vi "PLL_PID.vi"(8 "error in (no error)":errorcluster, 11 "DSP.lvclass":refnum<class "DSP.lvclass">) -> (0 "error out":errorcluster, 2 "phase out":dbl, 3 "DSP.lvclass":refnum<class "DSP.lvclass">)   [LabVIEW 2019, in "DSP.lvclass"]
uses:
  DSP.lvclass
  DSP.lvclass/DSP.ctl
  <vilib>/Analysis/baseanly.llb/Mean (DBL).vi
  <vilib>/addons/control/pid/pid.llb/PID (DBL).vi
  <vilib>/addons/control/pid/NI_PID_pid.lvlib
  <vilib>/Analysis/NI_AALBase.lvlib
panel:
  in  "x":dbl=4.77
  in  "mean?":bool
  out "TC (s)":dbl
  out "frequency (Hz)":dbl
  in  "PID gains (Phase)":T1={"proportional gain (Kc)"=-1.0, "integral time (Ti, min)"=0.025, "derivative time (Td, min)"=0.0} {"derivative time (Td, min)" format="%.3f"; "integral time (Ti, min)" format="%.3f"; "proportional gain (Kc)" format="%.3f"}
  out "Waveform Chart":T2(graph)
  # "4.77"
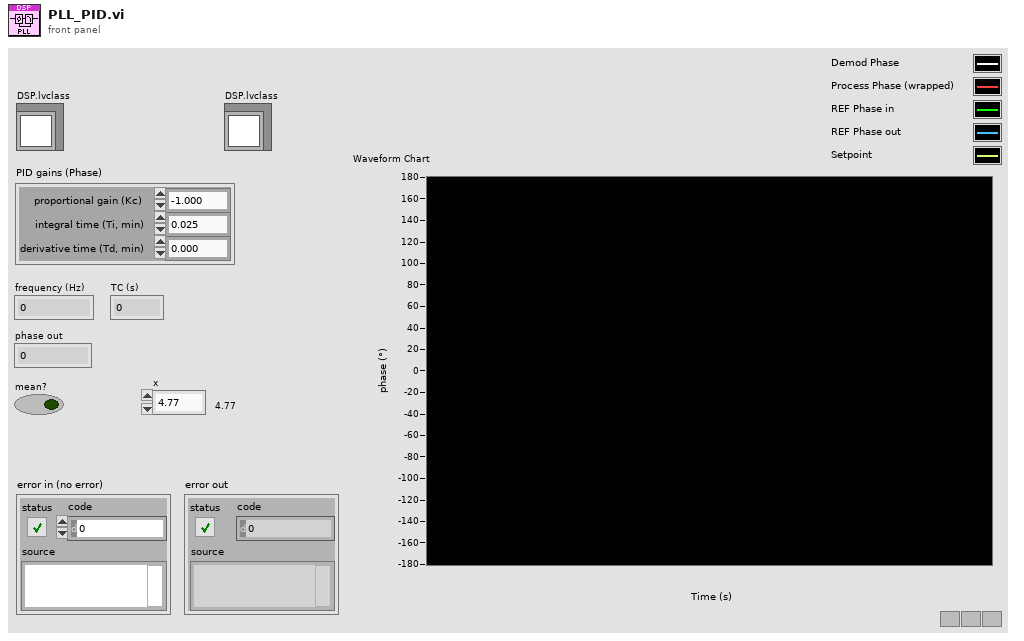
[diagram p1: front panel]
types:
  T1 = cluster{"proportional gain (Kc)":dbl, "integral time (Ti, min)":dbl, "derivative time (Td, min)":dbl}
  T2 = cluster{"value":dbl, "wrapped phase":dbl, "Phase":dbl, "wrapped phase":dbl, "setpoint":dbl}
  T3 = typedef "DSP.lvclass/REF.Channel--Cluster--Array.ctl" = T4[]
  T4 = typedef "DSP.lvclass/REF.Channel--Cluster.ctl" = cluster{"Enable?":bool, "Channel":i32, "Frequency":dbl, "Phase":dbl, "TC":dbl, "Roll-Off":i32}
  T5 = cluster{"value":dbl, "wrapped phase":dbl, "Phase":dbl, "wrapped phase":dbl, "setpoint":dbl}[]
  T6 = cluster{"filter structure":enum32{"IIR 2nd Order", "IIR 4th Order"}, "Reverse Coefficients":dbl[], "Forward Coefficients":dbl[]}[]
  T7 = cluster{dbl, "wrapped phase":dbl, "Phase":dbl, "wrapped phase":dbl, "setpoint":dbl}
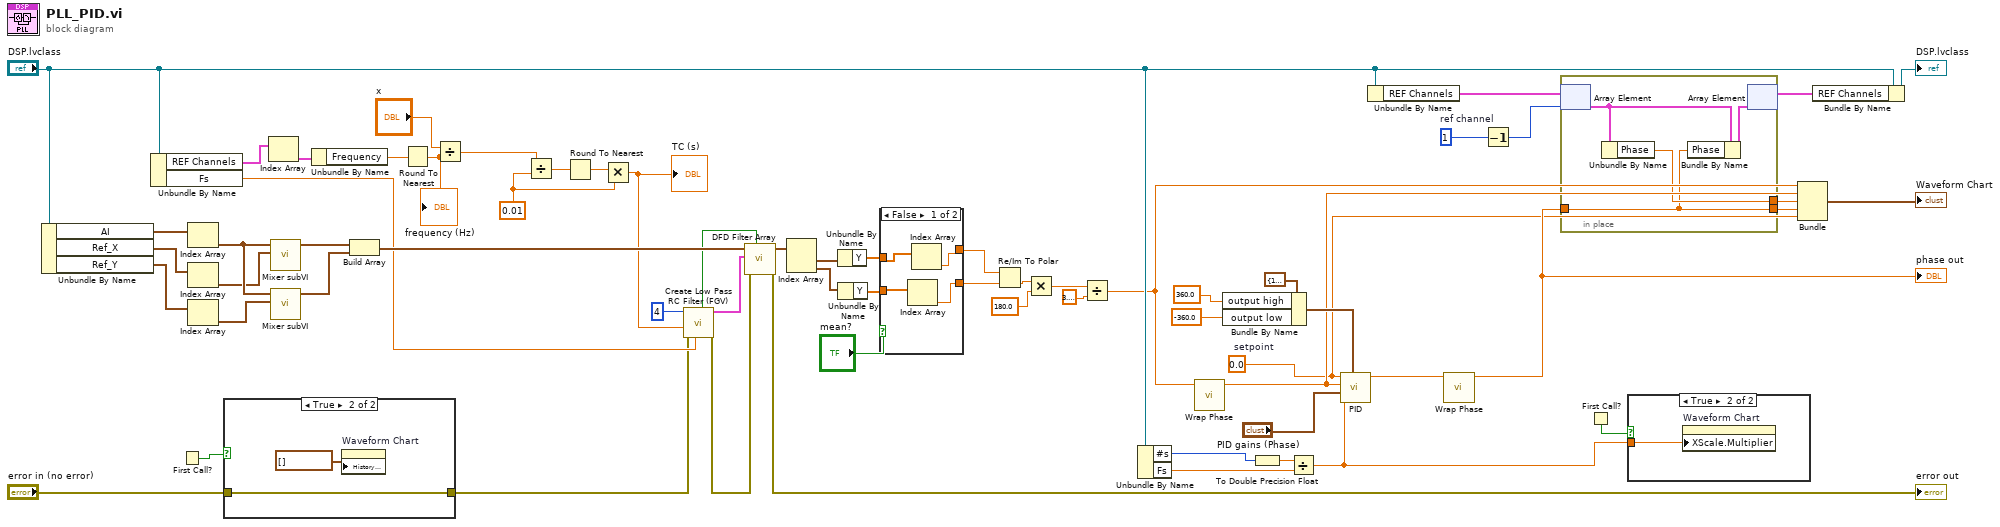
[diagram p0: block diagram]
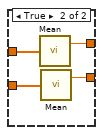
[diagram p2: hidden frame]
diagram:
  w2 = 0.01 ("y")
  w60 = 1  # ref channel
  w43 = 0.0  # setpoint
  n1 = Unbundle By Name("DSP.lvclass") -> ("AI"=w19:waveform(dbl)[], "Ref_X"=w17:waveform(dbl)[], "Ref_Y"=w16:waveform(dbl)[])
  n2 = Unbundle By Name("DSP.lvclass") -> ("REF Channels"=w36:T3, "Fs"=w37:dbl)
  n3 = First Call?() -> (First Call?: T/F=w46:bool)
  n4 = Index Array(array=w19) -> (element=w18:waveform(dbl))  [unwired: 1 in]
  n5 = Index Array(array=w17) -> (element=w15:waveform(dbl))  [unwired: 1 in]
  n6 = Index Array(array=w16) -> (element=w14:waveform(dbl))  [unwired: 1 in]
  n7 = case shown="True" w46 {
    tunnel: "error in (no error)" -> [w65 w66]
    tunnel: [w65 w66] -> w12
    frame False {
    }
    frame True {
      n8 = property on="Waveform Chart" class="WFChart (strict)"("History Data"=T5 []) -> ()  [unwired: 2 in, 2 out]
    }
  }
  n9 = Index Array(array=w36) -> (element=w35:T4)  [unwired: 1 in]
  n10 = call "Mixer subVI.vi"("Reference in"=w15, "Signal in"=w18) -> ("Signal*Reference out"=w41:waveform(dbl))  [unwired: 9 in]
  n11 = call "Mixer subVI.vi"("Reference in"=w14, "Signal in"=w18) -> ("Signal*Reference out"=w32:waveform(dbl))  [unwired: 9 in]
  n12 = Unbundle By Name(w35) -> ("Frequency"=w30:dbl)
  n13 = Build Array(w41, w32) -> (w40:waveform(dbl)[])
  n14 = Round To Nearest(number=w30) -> (nearest integer value=w29:dbl)
  "frequency (Hz)" <- w29
  n15 = Divide(x="x", y=w29) -> (x/y=w5:dbl)
  n16 = Divide(x=w5, y=w2) -> (x/y=w4:dbl)
  n17 = Round To Nearest(number=w4) -> (nearest integer value=w3:dbl)
  n18 = Multiply(x=w3, y=w2) -> (x*y=w1:dbl)
  "TC (s)" <- w1
  n19 = call "Create Low Pass RC Filter (FGV).vi"("fs (Hz)"=w37, "error in (no error)"=w12, "time constant (s)"=w1, "stages"=4 ("order")) -> ("error out"=w38:errorcluster, "IIR Filters"=w34:T6, "init out"=w39:bool)  [unwired: 5 in]
  n20 = call "DFD Filter Array.vi"("init (F)"=w39, "error in (no error)"=w38, "IIR Filters"=w34, "signal in"=w40) -> ("error out"=→"error out":errorcluster, "signal out"=w31:waveform(dbl)[])  [unwired: 6 in]
  n21 = Index Array(array=w31) -> (element #1=w22:waveform(dbl), element #2=w21:waveform(dbl))  [unwired: 2 in]
  n22 = Unbundle By Name(w22) -> ("Y"=w24:dbl[])
  n23 = Unbundle By Name(w21) -> ("Y"=w23:dbl[])
  n24 = case shown="False" "mean?" {
    tunnel: w24 -> [w69 w75]
    tunnel: w23 -> [w71 w74]
    tunnel: [w70 w73] -> w9
    tunnel: [w68 w72] -> w8
    frame False {
      n25 = Index Array(array=w71) -> (element=w70:dbl)  [unwired: 1 in]
      n26 = Index Array(array=w69) -> (element=w68:dbl)  [unwired: 1 in]
    }
    frame True {
      n27 = call-poly <vilib>:"Mean.vi"("X"=w75) -> ("mean"=w72:dbl)  [unwired: 1 out]
      n28 = call-poly <vilib>:"Mean.vi"("X"=w74) -> ("mean"=w73:dbl)  [unwired: 1 out]
    }
  }
  n29 = Re/Im To Polar(2:w9, 3:w8) -> (0:w26:dbl)  [unwired: 1 out]
  n30 = Multiply(x=w26, y=180.0) -> (x*y=w25:dbl)
  n31 = Divide(x=w25, y=3.141592653589793) -> (x/y=w11:dbl)
  n32 = Unbundle By Name("DSP.lvclass") -> ("#s"=w49:i32, "Fs"=w48:dbl)
  n33 = call "Wrap Phase.vi"("input phase"=w11) -> ("wrapped phase"=w47:dbl)  [unwired: 10 in]
  n34 = Bundle By Name(cluster=cluster{"output high":dbl, "output low":dbl} {"output high"=100.0, "output low"=-100.0} ("output range"), "output high"=360.0, "output low"=-360.0) -> (w62:cluster{"output high":dbl, "output low":dbl})
  n35 = To Double Precision Float(number=w49) -> (double precision float=w63:dbl)
  n36 = Divide(x=w63, y=w48) -> (x/y=w45:dbl)
  n37 = call-poly <vilib>:"PID.vi"("output range"=w62, "dt (s)"=w45, "PID gains"="PID gains (Phase)", "process variable"=w47, "setpoint"=w43) -> ("output"=w52:dbl)  [unwired: 5 in, 1 out]
  n38 = Unbundle By Name("DSP.lvclass") -> ("REF Channels"=w61:T3)
  n39 = call "Wrap Phase.vi"("input phase"=w52) -> ("wrapped phase"=w51:dbl)  [unwired: 10 in]
  "phase out" <- w51
  n40 = Decrement(x=w60) -> (x-1=w59:i32)
  n41 = in-place {
    in-place-border: w51 -> [w77]
    in-place-border: [w78] -> w57
    in-place-border: [w77] -> w56
    n42 = in-place-array #1(w61, w59) -> (w76:T4)
    n43 = Unbundle By Name(w76) -> ("Phase"=w78:dbl)
    n44 = Bundle By Name(cluster=w76, "Phase"=w77) -> (w79:T4)
    n45 = in-place-array #1(w79) -> (w58:T3)  [unwired: 1 out]
  }
  n46 = First Call?() -> (First Call?: T/F=w44:bool)
  n47 = case shown="True" w44 {
    tunnel: w45 -> [_ w80]
    frame False {
    }
    frame True {
      n48 = property on="Waveform Chart" class="WFChart (strict)"("XScale.Multiplier"=w80) -> ()  [unwired: 2 in, 2 out]
    }
  }
  n49 = Bundle(w11, "wrapped phase"=w47, "Phase"=w57, "wrapped phase"=w56, "setpoint"=w43) -> (→"Waveform Chart":T7)  [unwired: 1 in]
  n50 = Bundle By Name(cluster="DSP.lvclass", "REF Channels"=w58) -> (→"DSP.lvclass":refnum<class "DSP.lvclass">)
